vi "Apply DSF Configuration.vi"(8 "error in (no error)":errorcluster, 9 "version":T1, 10 "framework configuration":T2, 11 "Item Ref in":T18 format="%.0x") -> (0 "error out":errorcluster)   [LabVIEW 2020, in "DSF System Explorer.lvlib"]
uses:
  DSF System Explorer.lvlib
  <vilib>/NI VeriStand/Custom Device API/Custom Device Item Ref.ctl
  DSF Core.lvlibp/Typedefs/DSF Engine Framework Configuration.ctl
  DSF Core.lvlibp/Typedefs/DSF Engine Plugin Configuration.ctl
  DSF Core.lvlibp/Typedefs/Core Plugin Configuration.ctl
  DSF Core.lvlibp/Typedefs/DSF Timing Info.ctl
  DSF Core.lvlibp/Typedefs/DSF Settings Info.ctl
  DSF Core.lvlibp/Typedefs/DSF Engine Plugin Thread Configuration.ctl
  DSF Core.lvlibp/Typedefs/Core Thread Configuration.ctl
  DSF Core.lvlibp/Typedefs/DSF Engine Transfer Group Configuration.ctl
  DSF Core.lvlibp/Typedefs/Core Group Configuration.ctl
  DSF Core.lvlibp/Typedefs/DSF Direction.ctl
  DSF Core.lvlibp/Typedefs/DSF Timeout Behavior.ctl
  DSF Core.lvlibp/Typedefs/DSF Engine Transfer Configuration.ctl
  DSF Core.lvlibp/Typedefs/Core Transfer Configuration.ctl
  DSF Core.lvlibp/Typedefs/DSF Engine Channel Configuration.ctl
  DSF Core.lvlibp/Typedefs/Core Channel Configuration.ctl
  DSF Core.lvlibp/Typedefs/DSF Data Type.ctl
  DSF Core.lvlibp/Typedefs/DSF Version Info.ctl
  <vilib>/NI VeriStand/Custom Device API/NI VeriStand - Set Item Property.vi
  <vilib>/NI VeriStand/Custom Device API/Set Item Property (Variant).vi
  DSF Core.lvlibp/Classes/Configuration/Core/Framework/Framework Configuration.lvclass
  Source/DSF Core.lvlibp
  DSF Core.lvlibp/Classes/Configuration/Core/Plugin/Plugin Configuration.lvclass
  DSF Core.lvlibp/Classes/Configuration/Core/Thread/Thread Configuration.lvclass
  DSF Core.lvlibp/Classes/Configuration/Core/Group/Group Configuration.lvclass
  DSF Core.lvlibp/Classes/Configuration/Core/Transfer/Transfer Configuration.lvclass
  DSF Core.lvlibp/Classes/Configuration/Core/Channel/Channel Configuration.lvclass
  <vilib>/NI VeriStand/Custom Device API/Custom Device API.lvlib
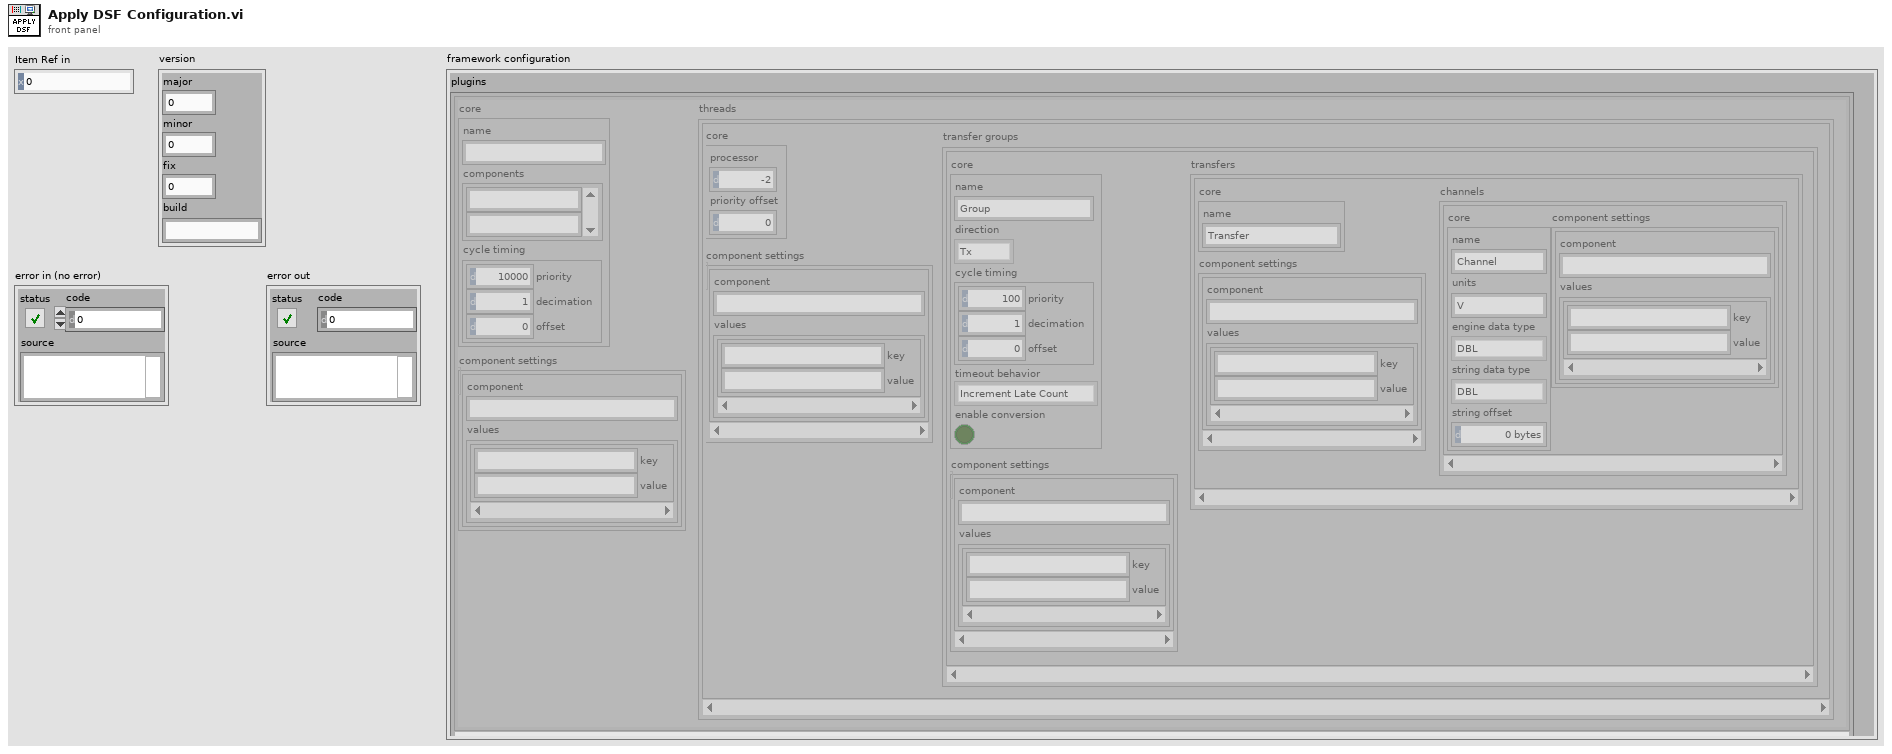
[diagram p1: front panel]
types:
  T1 = typedef "DSF Core.lvlibp/DSF Version Info.ctl" = cluster{"major":u32, "minor":u32, "fix":u32, "build":string}
  T2 = typedef "DSF Core.lvlibp/DSF Engine Framework Configuration.ctl" = cluster{"plugins":T3[]}
  T3 = typedef "DSF Core.lvlibp/DSF Engine Plugin Configuration.ctl" = cluster{"core":T4, "component settings":T6[], "threads":T7[]}
  T4 = typedef "DSF Core.lvlibp/Plugin Configuration.lvclass/Core Plugin Configuration.ctl" = cluster{"name":string, "components":string[], "cycle timing":T5}
  T5 = typedef "DSF Core.lvlibp/DSF Timing Info.ctl" = cluster{"priority":u64, "decimation":u64, "offset":u64}
  T6 = typedef "DSF Core.lvlibp/DSF Settings Info.ctl" = cluster{"component":string, "values":cluster{"key":string, "value":string}[]}
  T7 = typedef "DSF Core.lvlibp/DSF Engine Plugin Thread Configuration.ctl" = cluster{"core":T8, "component settings":T6[], "transfer groups":T9[]}
  T8 = typedef "DSF Core.lvlibp/Thread Configuration.lvclass/Core Thread Configuration.ctl" = cluster{"processor":i32, "priority offset":i16}
  T9 = typedef "DSF Core.lvlibp/DSF Engine Transfer Group Configuration.ctl" = cluster{"core":T10, "component settings":T6[], "transfers":T13[]}
  T10 = typedef "DSF Core.lvlibp/Group Configuration.lvclass/Core Group Configuration.ctl" = cluster{"name":string, "direction":T11, "cycle timing":T5, "timeout behavior":T12, "enable conversion":bool}
  T11 = typedef "DSF Core.lvlibp/DSF Direction.ctl" = enum8{"Tx", "Rx"}
  T12 = typedef "DSF Core.lvlibp/DSF Timeout Behavior.ctl" = enum8{"Increment Late Count", "Throw Error"}
  T13 = typedef "DSF Core.lvlibp/DSF Engine Transfer Configuration.ctl" = cluster{"core":T14, "component settings":T6[], "channels":T15[]}
  T14 = typedef "DSF Core.lvlibp/Transfer Configuration.lvclass/Core Transfer Configuration.ctl" = cluster{"name":string}
  T15 = typedef "DSF Core.lvlibp/DSF Engine Channel Configuration.ctl" = cluster{"core":T16, "component settings":T6[]}
  T16 = typedef "DSF Core.lvlibp/Channel Configuration.lvclass/Core Channel Configuration.ctl" = cluster{"name":string, "units":string, "engine data type":T17, "string data type":T17, "string offset":u64}
  T17 = typedef "DSF Core.lvlibp/DSF Data Type.ctl" = enum8{"Bool", "SGL", "DBL", "I8", "I16", "I32", "I64", "U8", "U16", "U32", "U64"}
  T18 = typedef "Custom Device API.lvlib/Custom Device Item Ref.ctl" = u64
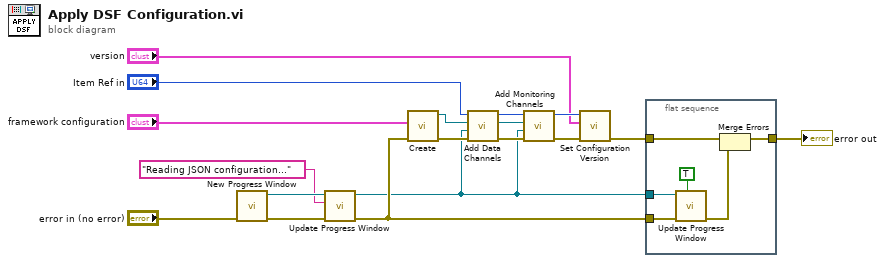
[diagram p0: block diagram]
diagram:
  n1 = call "New Progress Window.vi"("error in (no error)"="error in (no error)") -> ("error out"=w15:errorcluster, "progress queue"=w14:refnum<queue>)  [unwired: 9 in]
  n2 = call "Update Progress Window.vi"("error in (no error)"=w15, "message (\"\")"="Reading JSON configuration..." ("message"), "progress queue in"=w14) -> ("error out"=w6:errorcluster, "progress queue out"=w5:refnum<queue>)  [unwired: 7 in]
  n3 = call "Create.vi"("error in (no error)"=w6, "framework configuration"="framework configuration") -> ("error out"=w9:errorcluster, "Framework Configuration out"=w8:refnum<class "Framework Configuration.lvclass">)  [unwired: 8 in]
  n4 = call "Add Data Channels.vi"("error in (no error)"=w9, "progress queue"=w5, "Framework Configuration"=w8, "Item Ref in"="Item Ref in") -> ("error out"=w11:errorcluster, "Item Ref out"=w17:T18)  [unwired: 6 in]
  n5 = call "Add Monitoring Channels.vi"("error in (no error)"=w11, "progress queue"=w5, "Framework Configuration"=w8, "Item Ref in"=w17) -> ("error out"=w4:errorcluster, "Item Ref out"=w2:T18)  [unwired: 6 in]
  n6 = call "Set Configuration Version.vi"("error in (no error)"=w4, "version"="version", "Item Ref in"=w2) -> ("error out"=w3:errorcluster)  [unwired: 7 in, 1 out]
  n7 = flat-sequence {
    tunnel: w3 -> [w23]
    tunnel: [w21] -> w16
    tunnel: w6 -> [w19]
    tunnel: w5 -> [w18]
    frame #0 {
      n8 = call "Update Progress Window.vi"("stop (F)"=TRUE, "error in (no error)"=w19, "progress queue in"=w18) -> ("error out"=w22:errorcluster)  [unwired: 7 in, 1 out]
      n9 = Merge Errors(w23, w22) -> (w21:errorcluster)
    }
  }
  "error out" <- w16
